vi "LinearSystemId_IdentifyPositionSystem.vi"(10 "kA":dbl, 11 "kV":dbl) -> (3 "Linearsystem":T1)   [LabVIEW 2019, in "Trajectory_Library.lvlib"]
doc: "Creates a new LINEAR SYSTEM data cluster with the specified values. \n\n\nInputs: \n - XXX -- XXX.\n\nOutputs:\n - XXX -- XXX."
uses:
  Trajectory_Library.lvlib
  <vilib>/Analysis/Matrix/Datatypes/RealMatrix.ctl
  <vilib>/Analysis/Matrix/NI_Matrix.lvlib
  LINEAR_SYSTEM.ctl
panel:
  in  "Outputs":i32=1
  in  "Inputs":i32=1
  in  "States":i32=2
  # "<States,States>"
  # "<States,Inputs>"
  # "<Outputs,States>"
  # "<Outputs,Inputs>"
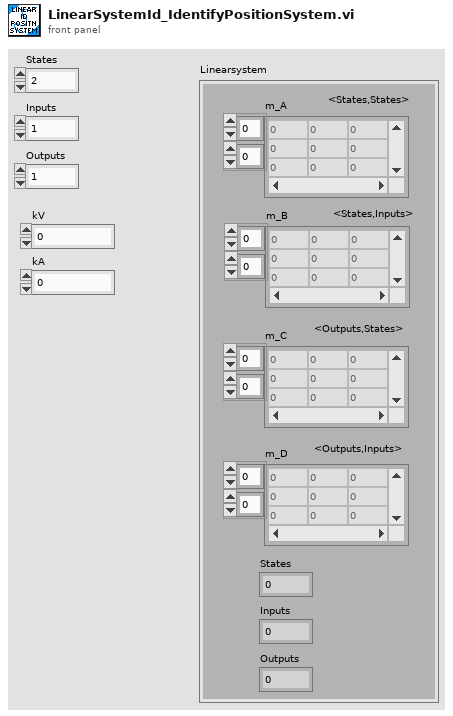
[diagram p1: front panel]
types:
  T1 = typedef "Trajectory_Library.lvlib/LINEAR_SYSTEM.ctl" = cluster{"m_A":T2, "m_B":T2, "m_C":T2, "m_D":T2, "States":i32, "Inputs":i32, "Outputs":i32}
  T2 = typedef "NI_Matrix.lvlib/RealMatrix.ctl" = dbl[][]
  T3 = typedef "Trajectory_Library.lvlib/LINEARSYSTEM.ctl" = cluster{"m_A":T2, "m_B":T2, "m_C":T2, "m_D":T2, "States":i32, "Inputs":i32, "Outputs":i32}
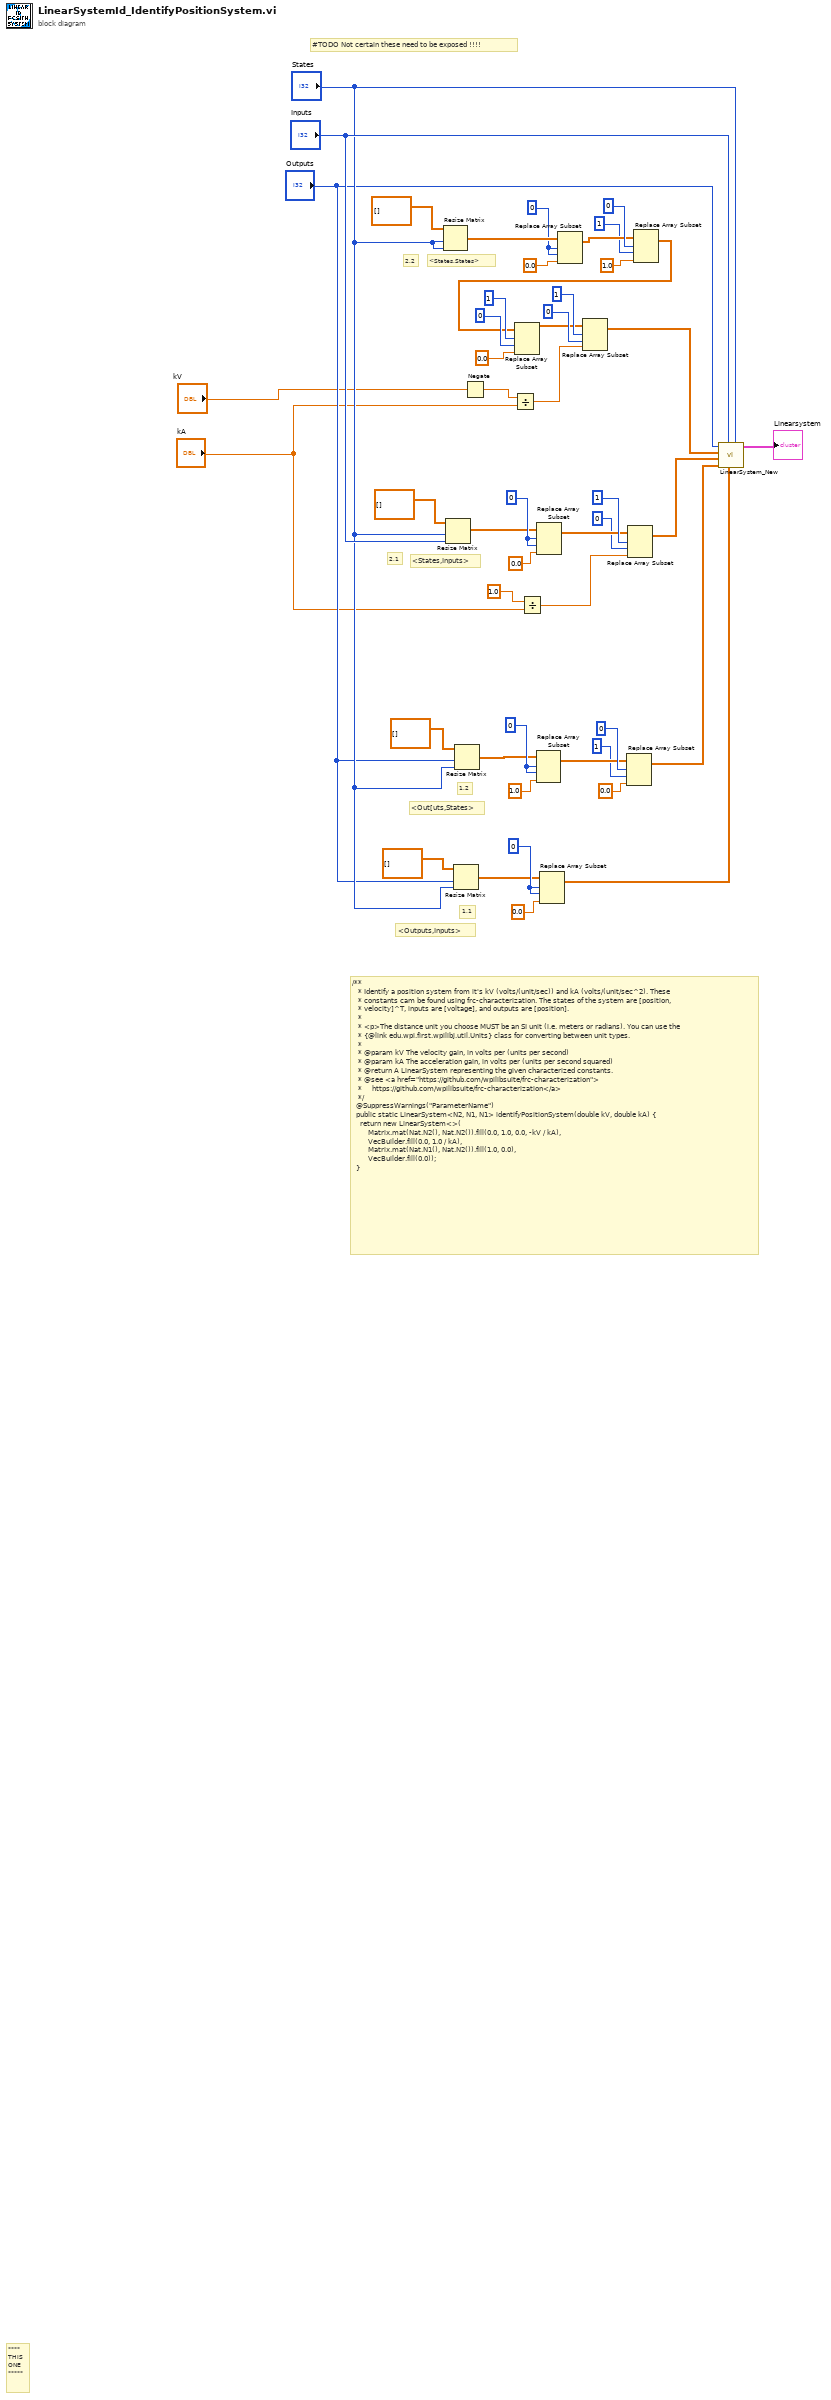
[diagram p0: block diagram]
diagram:
  w29 = 0 ("index (col)")
  w34 = 0 ("index (col)")
  w42 = 0 ("index (col)")
  w45 = 0 ("index (col)")
  # "2,2"
  # "2,1"
  # "1,2"
  # "1,1"
  # "<States,States>"
  # "<States,Inputs>"
  # "<Out[uts,States>"
  # "<Outputs,Inputs>"
  # "#TODO Not certain these need to be exposed !!!!"
  # "/**\n   * Identify a position system from it's kV (volts/(unit/sec)) and kA (volts/(unit/sec^2). These\n   * constants cam be found using frc-characterization. The states of the system are [position,\n   * velocity]^T, inputs are [voltage], and outputs are [position].\n   *\n   * <p>The distance unit you choose MUST be an SI unit (i.e. meters or radians). You can use the\n   * {@link edu.wpi.first.wpilibj.util.Units} class for converting between unit types.\n   *\n   * @param kV The velocity gain, in volts per (units per second)\n   * @param kA The acceleration gain, in volts per (units per second squared)\n   * @return A LinearSystem representing the given characterized constants.\n   * @see <a href=\"https://github.com/wpilibsuite/frc-characterization\">\n   *     https://github.com/wpilibsuite/frc-characterization</a>\n   */\n  @SuppressWarnings(\"ParameterName\")\n  public static LinearSystem<N2, N1, N1> identifyPositionSystem(double kV, double kA) {\n    return new LinearSystem<>(\n        Matrix.mat(Nat.N2(), Nat.N2()).fill(0.0, 1.0, 0.0, -kV / kA),\n        VecBuilder.fill(0.0, 1.0 / kA),\n        Matrix.mat(Nat.N1(), Nat.N2()).fill(1.0, 0.0),\n        VecBuilder.fill(0.0));\n  }"
  # "****\nTHIS\nONE\n*****"
  n1 = Resize Matrix(1:"States", 2:"States", 4:T2 [] ("matrix")) -> (0:w46:T2)
  n2 = Resize Matrix(1:"Inputs", 2:"States", 4:T2 [] ("matrix")) -> (0:w24:T2)
  n3 = Resize Matrix(1:"States", 2:"Outputs", 4:T2 [] ("matrix")) -> (0:w32:T2)
  n4 = Resize Matrix(1:"States", 2:"Outputs", 4:T2 [] ("matrix")) -> (0:w40:T2)
  n5 = Negate(x="kV") -> (-x=w3:dbl)
  n6 = Divide(x=w3, y="kA") -> (x/y=w6:dbl)
  n7 = Divide(x=1.0, y="kA") -> (x/y=w5:dbl)
  n8 = Replace Array Subset(array=w40, new element=1.0 ("new element/submatrix"), index (row)=w42, index (col)=w42) -> (w39:T2)
  n9 = Replace Array Subset(array=w24, new element=0.0 ("new element/submatrix"), index (row)=w29, index (col)=w29) -> (w27:T2)
  n10 = Replace Array Subset(array=w32, new element=0.0 ("new element/submatrix"), index (row)=w34, index (col)=w34) -> (w31:T2)
  n11 = Replace Array Subset(array=w46, new element=0.0 ("new element/submatrix"), index (row)=w45, index (col)=w45) -> (w18:T2)
  n12 = Replace Array Subset(array=w39, new element=0.0 ("new element/submatrix"), index (row)=0 ("index (col)"), index (col)=1 ("disabled index (col)")) -> (w38:T2)
  n13 = Replace Array Subset(array=w27, new element=w5, index (row)=1 ("index (col)"), index (col)=0 ("disabled index (col)")) -> (w23:T2)
  n14 = Replace Array Subset(array=w18, new element=1.0 ("new element/submatrix"), index (row)=0 ("index (col)"), index (col)=1 ("disabled index (col)")) -> (w11:T2)
  n15 = Replace Array Subset(array=w11, new element=0.0 ("new element/submatrix"), index (row)=1 ("index (col)"), index (col)=0 ("disabled index (col)")) -> (w12:T2)
  n16 = Replace Array Subset(array=w12, new element=w6, index (row)=1 ("index (col)"), index (col)=0 ("disabled index (col)")) -> (w10:T2)
  n17 = call "LinearSystem_New.vi"("States"="States", "D"=w31, "Inputs"="Inputs", "C"=w38, "B"=w23, "A"=w10, "Outputs"="Outputs") -> ("Linearsystem"=→"Linearsystem":T3)  [unwired: 4 in]
